vi "tcp_client_UI.vi"(10 "软件升级":refnum<vi>, 11 "data":refnum<vi>) -> ()   [LabVIEW 2016, in "数据传输系统-05.lvlib" / "update.lvlib"]
uses:
  update.lvlib
  tcp_client_data.ctl
  TCP_client/TCP_client.lvclass
  TCP_client/TCP_client.lvclass/TCP_client.ctl
panel:
  out "read":string
  in  "服务器信息":cluster{"host":string, "port":u16}={"host"="121.36.219.111", "port"=10001}
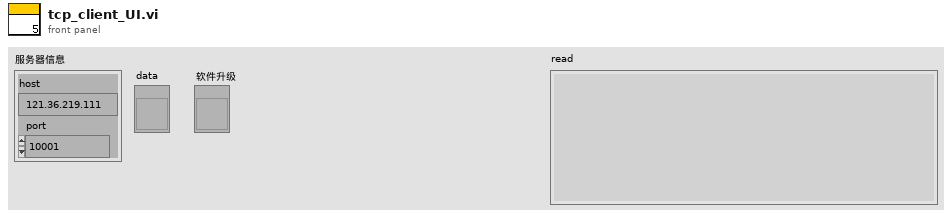
[diagram p1: front panel]
types:
  T1 = typedef "update.lvlib/tcp_client_data.ctl" = cluster{"SPname":string, "MNnumber":string, "Version":string, "state":string, "progress":dbl, "password":string, "data_transmission_Version":string}
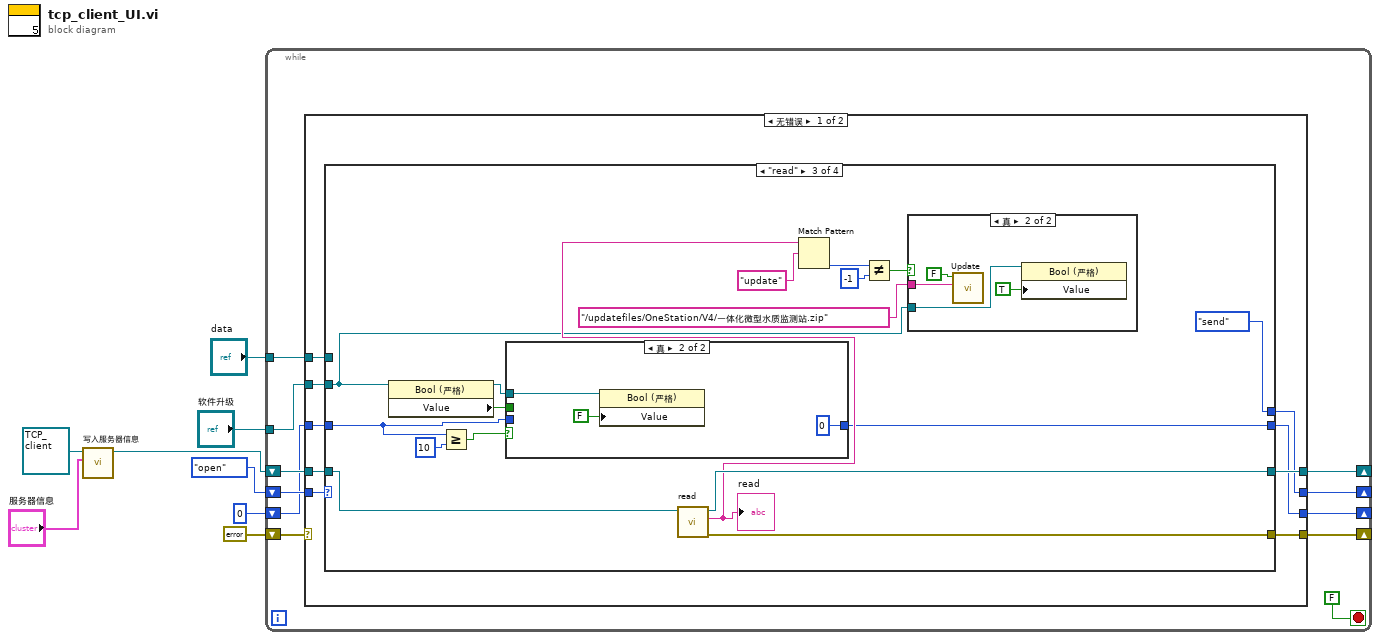
[diagram p0: block diagram]
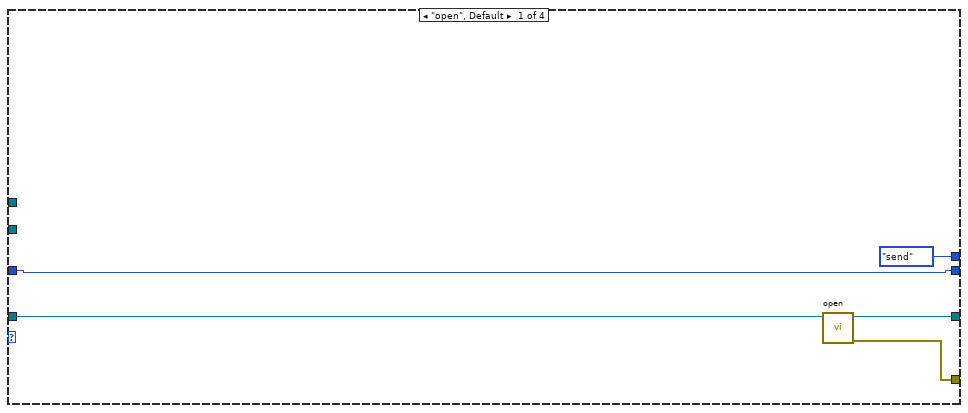
[diagram p2: hidden frame]
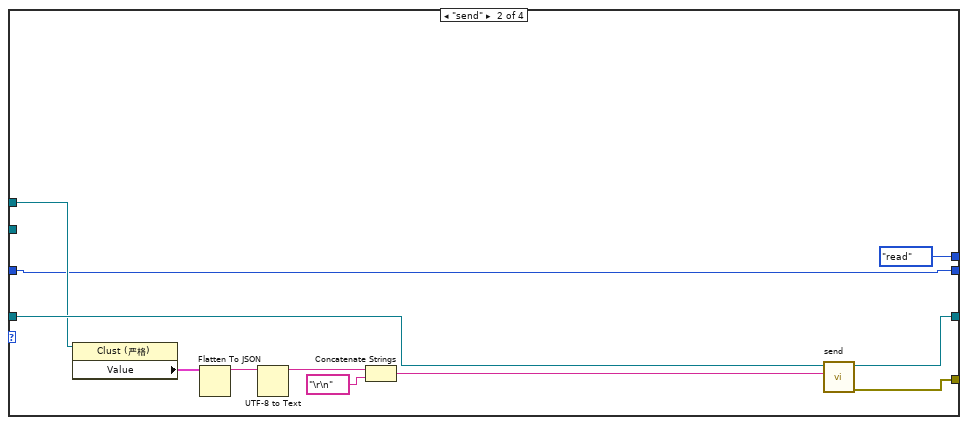
[diagram p3: hidden frame]
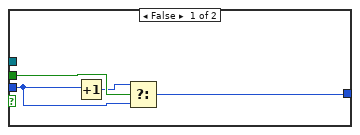
[diagram p4: hidden frame]
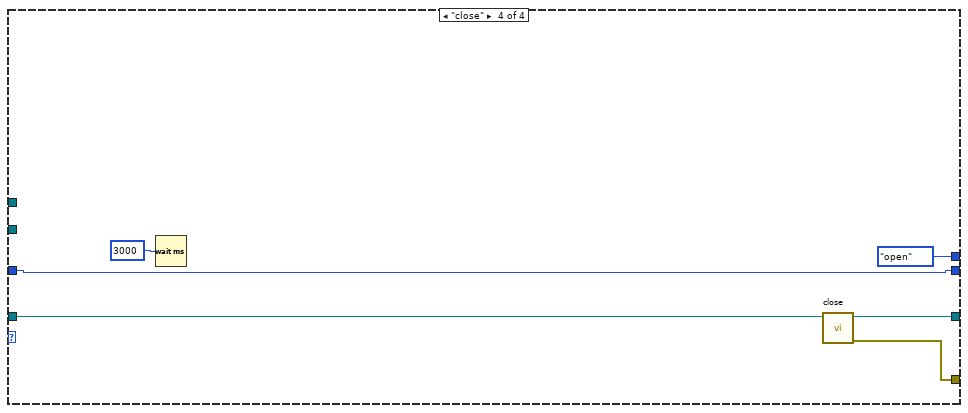
[diagram p6: hidden frame]
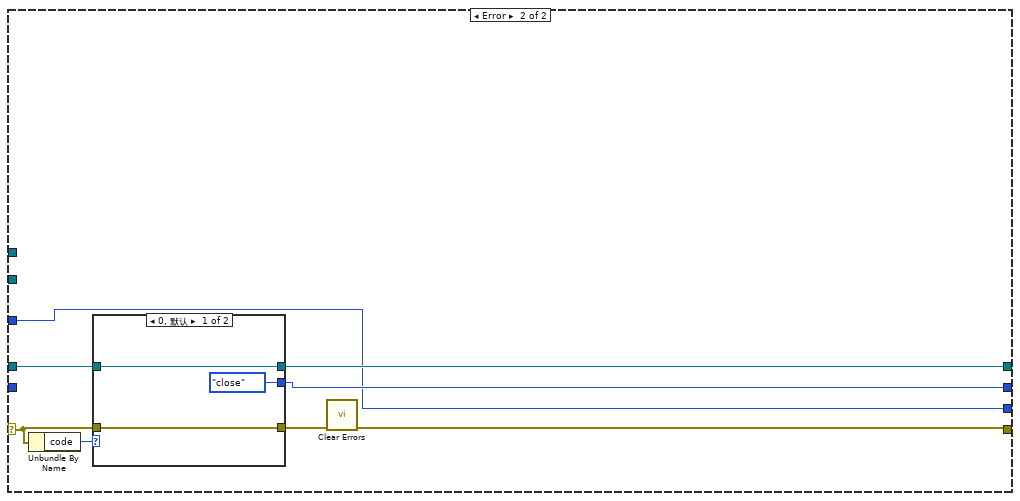
[diagram p7: hidden frame]
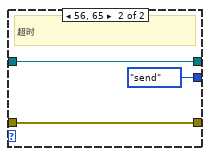
[diagram p8: hidden frame]
diagram:
  n1 = call "写入服务器信息.vi"("服务器信息"="服务器信息", "TCP_client输入"=refnum<class "TCP_client.lvclass"> refnum ("TCP_client.lvclass")) -> ("TCP_client输出"=w6:refnum<class "TCP_client.lvclass">)  [unwired: 8 in, 1 out]
  n2 = while {
    shift-right: [w13] -> _
    shift-left: enum16{"open", "send", "read", "close"}."open" -> [w18]
    shift-right: [w16] -> _
    shift-left: errorcluster {"status"=FALSE, "code"=0, "source"=""} ("error out") -> [w15]
    shift-right: [w14] -> _
    shift-left: w6 -> [w19]
    tunnel: "data" -> [w12]
    tunnel: "软件升级" -> [w11]
    shift-right: [w9] -> _
    shift-left: 0 -> [w10]
    stop <- FALSE stop-if-true
    n3 = case shown="无错误" w15 {
      selector: w15 -> [_ w83]
      tunnel: w19 -> [w28 w85]
      tunnel: w18 -> [w27 _]
      tunnel: [w26 w80] -> w16
      tunnel: [w25 w84] -> w14
      tunnel: [w24 w82] -> w13
      tunnel: w12 -> [w23 _]
      tunnel: w11 -> [w22 _]
      tunnel: w10 -> [w21 w79]
      tunnel: [w20 w79] -> w9
      frame No Error {
        n4 = case shown="\"read\"" w27 {
          tunnel: w28 -> [w33 w44 w61 w78]
          tunnel: [w32 w43 w59 w77] -> w26
          tunnel: [w31 w42 w60 w76] -> w25
          tunnel: [enum16{"open", "send", "read", "close"}."send" enum16{"open", "send", "read", "close"}."read" enum16{"open", "send", "read", "close"}."send" enum16{"open", "send", "read", "close"}."open"] -> w24
          tunnel: w23 -> [_ w38 _ _]
          tunnel: w22 -> [_ _ w51 _]
          tunnel: w21 -> [w29 w34 w46 w73]
          tunnel: [w29 w34 w49 w73] -> w20
          frame "open", Default {
            n5 = call-dynamic "open.vi"("TCP_client 输入"=w33) -> ("error out"=w32:errorcluster, "TCP_client 输出"=w31:refnum<class "TCP_client.lvclass">)  [unwired: 9 in]
          }
          frame "send" {
            n6 = property class="Clust (严格)"(reference=w38) -> ("Value"=w35:T1)  [unwired: 1 in, 2 out]
            n7 = Flatten To JSON(anything=w35) -> (JSON string=w37:string)  [unwired: 2 in, 1 out]
            n8 = UTF-8 to Text(11:w37) -> (3:w36:string)  [unwired: 2 in, 1 out]
            n9 = Concatenate Strings(w36, "\r\n" ("字符串")) -> (w39:string)
            n10 = call-dynamic "send.vi"("send"=w39, "TCP_client 输入"=w44) -> ("error out"=w43:errorcluster, "TCP_client 输出"=w42:refnum<class "TCP_client.lvclass">)  [unwired: 8 in]
          }
          frame "read" {
            n11 = property class="Bool (严格)"(reference=w51) -> (reference out=w45:refnum<vi>, "Value"=w50:bool)  [unwired: 1 in, 1 out]
            n12 = Greater Or Equal?(x=w46, y=10) -> (x >= y?=w47:bool)
            n13 = case shown="真" w47 {
              tunnel: w50 -> [w65 _]
              tunnel: [w63 0] -> w49
              tunnel: w46 -> [w62 _]
              tunnel: w45 -> [_ w67]
              frame False {
                n14 = Increment(x=w62) -> (x+1=w64:i32)
                n15 = Select(t=w64, s=w65, f=w62) -> (s? t:f=w63:i32)
              }
              frame True {
                n16 = property class="Bool (严格)"(reference=w67, "Value"=FALSE ("值")) -> ()  [unwired: 1 in, 2 out]
              }
            }
            n17 = call-dynamic "read.vi"("TCP_client 输入"=w61) -> ("error out"=w59:errorcluster, "read"=w57:string, "TCP_client 输出"=w60:refnum<class "TCP_client.lvclass">)  [unwired: 8 in]
            "read" <- w57
            n18 = Match Pattern(string=w57, regular expression="update" ("正则表达式")) -> (offset past match=w55:i32)  [unwired: 1 in, 3 out]
            n19 = Not Equal?(x=w55, y=-1) -> (x != y?=w52:bool)
            n20 = case shown="真" w52 {
              tunnel: "/updatefiles/OneStation/V4/一体化微型水质监测站.zip" ("更新包远端地址") -> [_ w72]
              tunnel: w51 -> [_ w70]
              frame False {
              }
              frame True {
                n21 = call "Update.vi"("更新包远端地址"=w72, "测试版？"=FALSE) -> ()  [unwired: 10 in]
                n22 = property class="Bool (严格)"(reference=w70, "Value"=TRUE ("值")) -> ()  [unwired: 1 in, 2 out]
              }
            }
          }
          frame "close" {
            n23 = Wait (ms)(milliseconds to wait=u32 3000 ("等待时间（毫秒）")) -> ()  [unwired: 1 out]
            n24 = call-dynamic "close.vi"("TCP_client 输入"=w78) -> ("error out"=w77:errorcluster, "TCP_client 输出"=w76:refnum<class "TCP_client.lvclass">)  [unwired: 9 in]
          }
        }
      }
      frame Error {
        n25 = Unbundle By Name(w83) -> ("code"=w86:i32)
        n26 = case shown="0, 默认" w86 {
          tunnel: w85 -> [w88 w92]
          tunnel: [w88 w92] -> w84
          tunnel: [w87 w90] -> w81
          tunnel: w83 -> [w87 w90]
          tunnel: [enum16{"open", "send", "read", "close"}."close" enum16{"open", "send", "read", "close"}."send"] -> w82
          frame 0, Default {
          }
          frame 56, 65 {
            # "超时"
          }
        }
        n27 = call <vilib>:"Clear Errors.vi"("error in (no error)"=w81) -> ("error out"=w80:errorcluster)  [unwired: 5 in, 1 out]
      }
    }
  }
